vi "ColorVariablesTC.vi"(8 "error in (no error)":errorcluster, 11 "VMUI in":refnum<class "VMUI.lvclass">=refnum) -> (0 "error out":errorcluster, 3 "VMUI out":refnum<class "VMUI.lvclass">)   [LabVIEW 2013, in "VMUI.lvclass"]
uses:
  VMUI.lvclass
  <vilib>/Utility/miscctls.llb/LVRowAndColumnTypeDef.ctl
  API/VariableManagerAPI.lvlib
panel:
  in  "ColorInd2":u32(colorbox)=13816530
  in  "ColorInd":u32(colorbox)=12910532
  in  "ColorFalse":u32(colorbox)=1985280
  in  "ColorTrue":u32(colorbox)=6618880
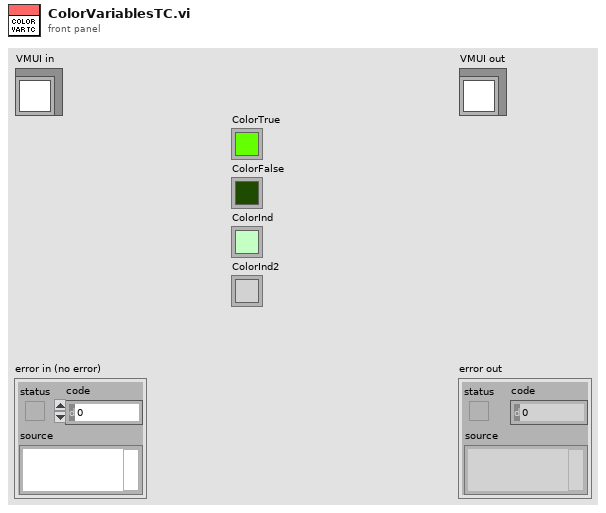
[diagram p1: front panel]
types:
  T1 = typedef "LVRowAndColumnTypeDef.ctl" = cluster{"Row":i32, "Column":i32}
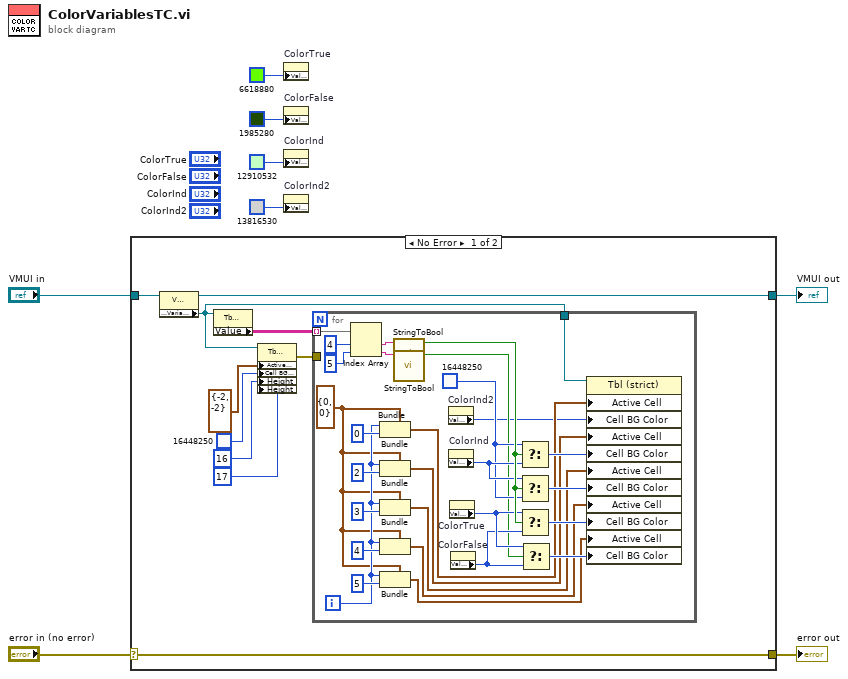
[diagram p0: block diagram]
diagram:
  n1 = case shown="No Error" "error in (no error)" {
    selector: "error in (no error)" -> [w18 w49]
    tunnel: [w18 w49] -> w7
    tunnel: [w16 w48] -> w5
    tunnel: "VMUI in" -> [w17 w48]
    frame No Error {
      n2 = property class="VMUI.lvclass"(reference=w17) -> (reference out=w16:refnum<class "VMUI.lvclass">, "Accessors:VariablesTCRef"=w12:refnum<vi>)  [unwired: 1 in, 1 out]
      n3 = property class="Tbl (strict)"(reference=w12) -> ("Value"=w14:string[][])  [unwired: 1 in, 2 out]
      n4 = property class="Tbl (strict)"(reference=w12, "Active Cell"=T1 {"Row"=-2, "Column"=-2} ("Active Cell:Active Cell"), "Cell BG Color"=u32 16448250, "Height"=u32 16 ("Active Cell:Cell Size:Height"), "Height"=u32 17 ("Active Cell:Cell Size:Height")) -> (error out=w13:errorcluster)  [unwired: 1 in, 1 out]
      n5 = for {
        tunnel: w14 -> [w45] mode=indexing
        tunnel: w12 -> [w25]
        tunnel: w13 -> [_]
        i -> [w37]
        w31 = u32 16448250
        w36 = T1 {"Row"=0, "Column"=0} ("Active Cell:Active Cell")
        n6 = Index Array(array=w45, index #1=4 ("index"), index #2=5 ("index")) -> (element #1=w43:string, element #2=w44:string)
        n7 = Bundle(cluster=w36, "Row"=w37, "Column"=0) -> (w24:T1)
        n8 = Bundle(cluster=w36, "Row"=w37, "Column"=2) -> (w23:T1)
        n9 = Bundle(cluster=w36, "Row"=w37, "Column"=3) -> (w22:T1)
        n10 = Bundle(cluster=w36, "Row"=w37, "Column"=4) -> (w21:T1)
        n11 = Bundle(cluster=w36, "Row"=w37, "Column"=5) -> (w20:T1)
        n12 = call "StringToBool.vi"("StringIn"=w43) -> ("Boolean"=w35:bool)  [unwired: 10 in]
        n13 = call "StringToBool.vi"("StringIn"=w44) -> ("Boolean"=w30:bool)  [unwired: 10 in]
        n14 = property on="ColorInd2" class="ColBox"() -> ("Value"=w19:u32)  [unwired: 2 in, 2 out]
        n15 = property on="ColorInd" class="ColBox"() -> ("Value"=w32:u32)  [unwired: 2 in, 2 out]
        n16 = property on="ColorTrue" class="ColBox"() -> ("Value"=w34:u32)  [unwired: 2 in, 2 out]
        n17 = property on="ColorFalse" class="ColBox"() -> ("Value"=w33:u32)  [unwired: 2 in, 2 out]
        n18 = Select(t=w31, s=w35, f=w32) -> (s? t:f=w29:u32)
        n19 = Select(t=w32, s=w35, f=w31) -> (s? t:f=w28:u32)
        n20 = Select(t=w34, s=w35, f=w33) -> (s? t:f=w27:u32)
        n21 = Select(t=w34, s=w30, f=w33) -> (s? t:f=w26:u32)
        n22 = property class="Tbl (strict)"(reference=w25, "Active Cell"=w24, "Cell BG Color"=w19, "Active Cell"=w23, "Cell BG Color"=w29, "Active Cell"=w22, "Cell BG Color"=w28, "Active Cell"=w21, "Cell BG Color"=w27, "Active Cell"=w20, "Cell BG Color"=w26) -> ()  [unwired: 1 in, 2 out]
      }
    }
    frame Error {
    }
  }
  "error out" <- w7
  "VMUI out" <- w5
  n23 = property on="ColorTrue" class="ColBox"("Value"=u32 6618880) -> ()  [unwired: 2 in, 2 out]
  n24 = property on="ColorFalse" class="ColBox"("Value"=u32 1985280) -> ()  [unwired: 2 in, 2 out]
  n25 = property on="ColorInd" class="ColBox"("Value"=u32 12910532) -> ()  [unwired: 2 in, 2 out]
  n26 = property on="ColorInd2" class="ColBox"("Value"=u32 13816530) -> ()  [unwired: 2 in, 2 out]
